vi "Modbus_spy.vi"() -> ()   [LabVIEW 2012]
uses:
  Controls/MBA_data.ctl
  <vilib>/Instr/_visa.llb/VISA Configure Serial Port (Instr).vi
panel:
  in  "string":string
  out "MBA data":T1
  in  "Array":string[](array[string])
  in  "Стоп":bool
  out "substring":string
  out "error out":errorcluster
  in  "error in (no error)":errorcluster
  in  "flow control":u16(ring) items=["None"=0, "XON/XOFF"=1, "RTS/CTS"=2, "DTR/DSR"=4]
  in  "stop bits":u16(ring)=10 items=["1.0"=10, "1.5"=15, "2.0"=20]
  in  "parity":u16(ring)=1 items=["None", "Odd", "Even", "Mark", "Space"]
  in  "data bits":u16=8 min=5 max=8 step=1
  in  "VISA resource name":refnum<visa-resource-name>="COM1"
  in  "baud rate":u32=19200
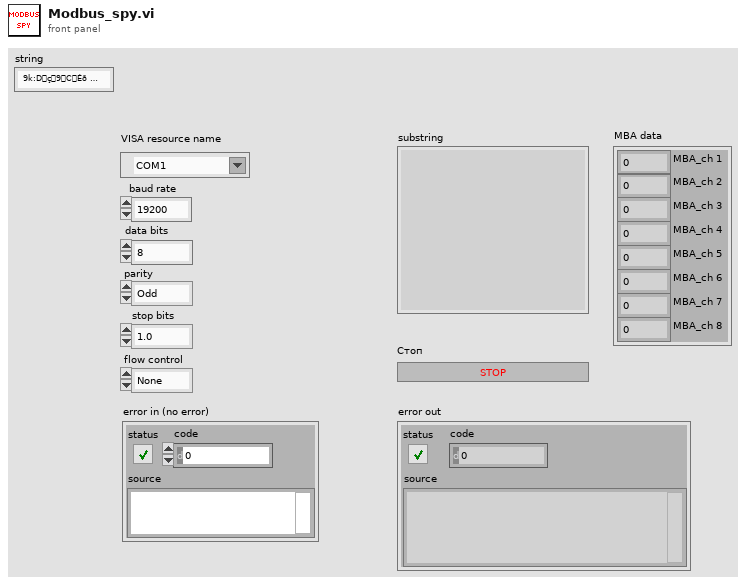
[diagram p1: front panel]
types:
  T1 = typedef "MBA_data.ctl" = cluster{"MBA_ch 1":dbl, "MBA_ch 2":dbl, "MBA_ch 3":dbl, "MBA_ch 4":dbl, "MBA_ch 5":dbl, "MBA_ch 6":dbl, "MBA_ch 7":dbl, "MBA_ch 8":dbl}
  T2 = cluster{"MBA_ch 1":dbl, "MBA_ch 2":dbl, "MBA_ch 3":dbl, "MBA_ch 4":dbl, "MBA_ch 5":dbl, "MBA_ch 6":dbl, "MBA_ch 7":dbl, "MBA_ch 8":dbl}
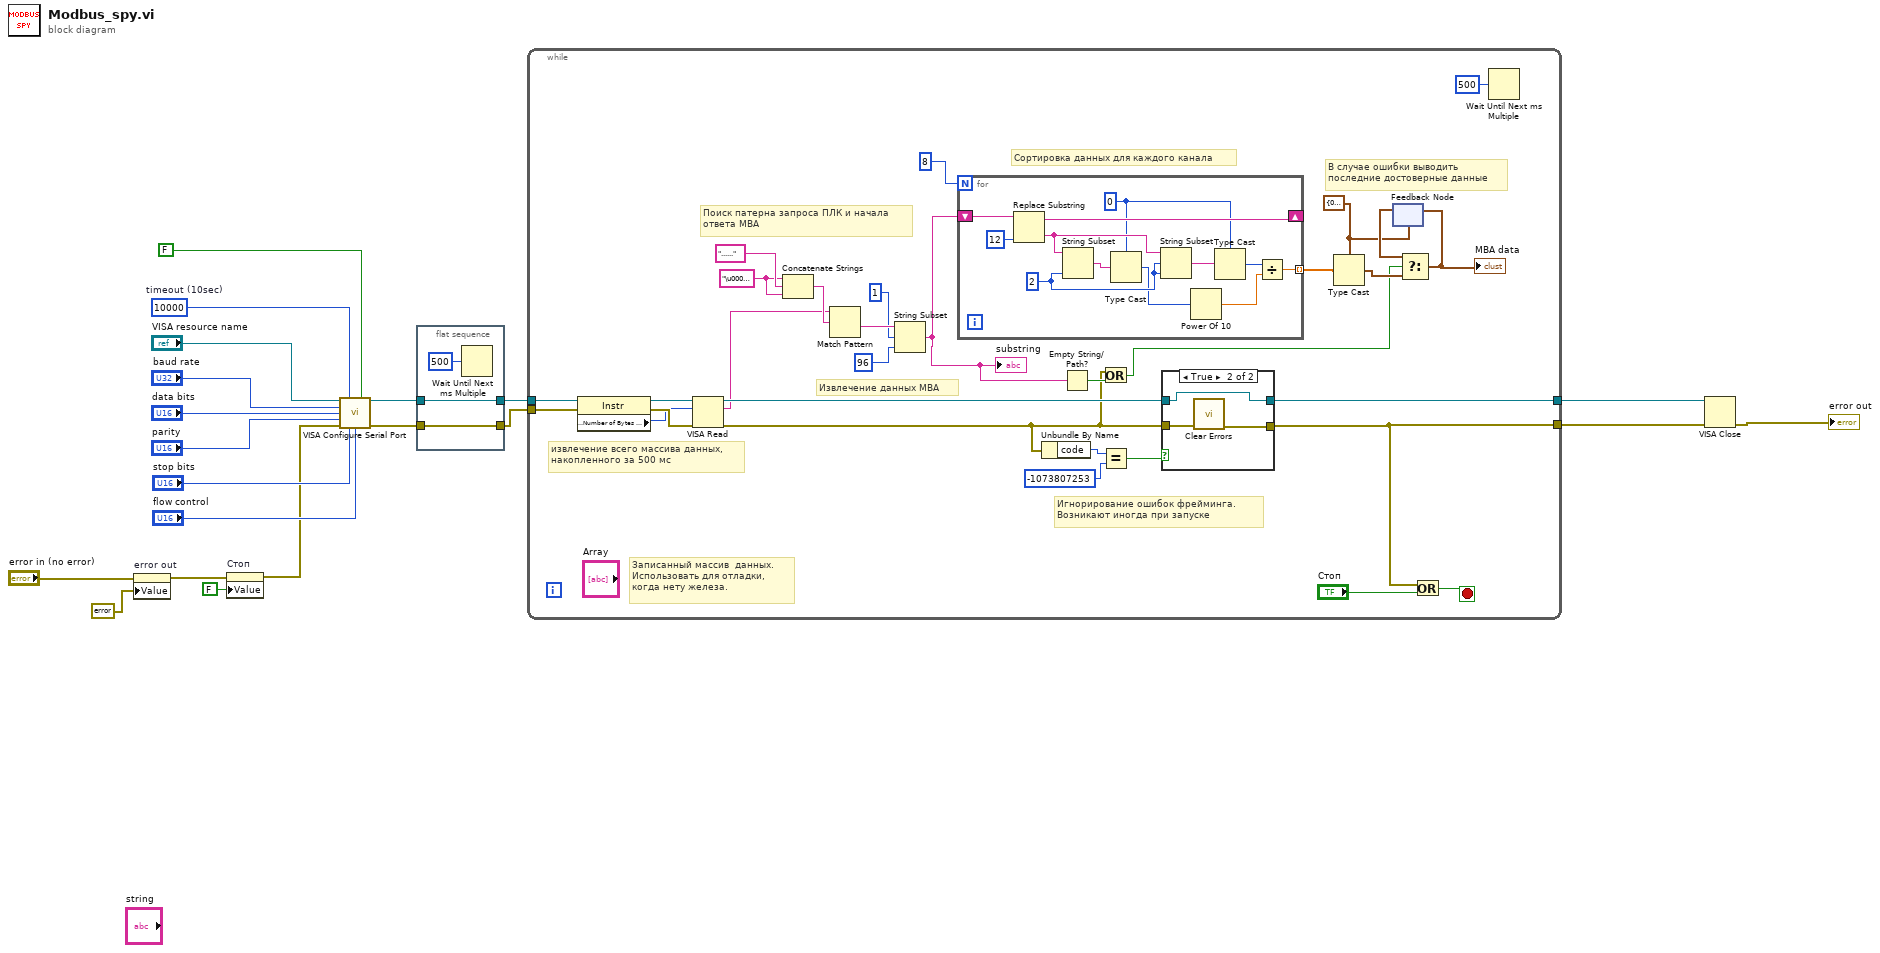
[diagram p0: block diagram]
diagram:
  w16 = u32 10000  # timeout (10sec)
  n1 = property on="error out" class="Clust (strict)"(error in="error in (no error)", "Value"=errorcluster {"status"=FALSE, "code"=0, "source"=""} ("error in (no error)")) -> (error out=w3:errorcluster)  [unwired: 1 in, 1 out]
  n2 = property on="Стоп" class="Bool (strict)"(error in=w3, "Value"=FALSE ("Стоп")) -> (error out=w6:errorcluster)  [unwired: 1 in, 1 out]
  n3 = call-poly "VISA Configure Serial Port"("VISA resource name"="VISA resource name", "timeout (10sec)"=w16, "Enable Termination\nChar (T)"=FALSE ("Enable Termination\nChar (T)"), "baud rate (9600)"="baud rate", "data bits (8)"="data bits", "parity (0:none)"="parity", "error in (no error)"=w6, "stop bits (10: 1 bit)"="stop bits", "flow control (0:none)"="flow control") -> ("VISA resource name out"=w10:refnum<visa-resource-name>, "error out"=w8:errorcluster)  [unwired: 5 out]
  n4 = flat-sequence {
    tunnel: w10 -> [w22]
    tunnel: [w22] -> w9
    tunnel: w8 -> [w21]
    tunnel: [w21] -> w7
    frame #0 {
      n5 = Wait Until Next ms Multiple(millisecond multiple=u32 500) -> ()  [unwired: 1 out]
    }
  }
  n6 = while {
    tunnel: [w32] -> w20
    tunnel: w9 -> [w51]
    tunnel: w7 -> [w50]
    tunnel: [w39] -> w4
    stop <- w45 stop-if-true
    w29 = T2 {"MBA_ch 1"=0.0, "MBA_ch 2"=0.0, "MBA_ch 3"=0.0, "MBA_ch 4"=0.0, "MBA_ch 5"=0.0, "MBA_ch 6"=0.0, "MBA_ch 7"=0.0, "MBA_ch 8"=0.0} ("MBA data")
    w48 = "\u0002\u0003" ("string")
    # "В случае ошибки выводить \nпоследние достоверные данные"
    # "Записанный массив  данных.\nИспользовать для отладки,\nкогда нету железа."
    # "Сортировка данных для каждого канала"
    # "Извлечение данных МВА"
    # "Игнорирование ошибок фрейминга.\nВозникают иногда при запуске"
    # "Поиск патерна запроса ПЛК и начала\nответа МВА"
    # "извлечение всего массива данных,\nнакопленного за 500 мс"
    n7 = property class="Instr"(reference=w51, error in=w50) -> (reference out=w54:refnum<visa-resource-name>, error out=w53:errorcluster, "Serial Settings:Number of Bytes at Serial Port"=w52:u32)
    n8 = VISA Read(VISA resource name=w54, byte count=w52, error in (no error)=w53) -> (VISA resource name out=w40:refnum<visa-resource-name>, read buffer=w33:string, error out=w25:errorcluster)  [unwired: 1 out]
    n9 = Concatenate Strings(w48, "......" ("regular expression"), w48) -> (w47:string)
    n10 = Match Pattern(string=w33, regular expression=w47) -> (after substring=w38:string)  [unwired: 1 in, 3 out]
    n11 = String Subset(string=w38, offset (0)=1, length (rest)=96 ("length (len. of substring)")) -> (substring=w27:string)
    "substring" <- w27
    n12 = for {
      N: 8 -> [_]
      shift-right: [w64] -> _
      shift-left: w27 -> [w66]
      tunnel: [w55] -> w34 mode=indexing
      w59 = i16 0
      w62 = 2 ("length (rest)")
      n13 = Replace Substring(2:12 ("length (len. of substring)"), 5:w66) -> (0:w61:string, 1:w64:string)  [unwired: 2 in]
      n14 = String Subset(string=w61, length (rest)=w62) -> (substring=w63:string)  [unwired: 1 in]
      n15 = Type Cast(type=w59, x=w63) -> (*(type *) &x=w57:i16)
      n16 = String Subset(string=w61, offset (0)=w62, length (rest)=w62) -> (substring=w60:string)
      n17 = Power Of 10(x=w57) -> (10^x=w56:dbl)
      n18 = Type Cast(type=w59, x=w60) -> (*(type *) &x=w58:i16)
      n19 = Divide(x=w58, y=w56) -> (x/y=w55:dbl)
    }
    n20 = Unbundle By Name(w25) -> ("code"=w43:i32)
    n21 = Empty String/Path?(string/path=w27) -> (empty?=w26:bool)
    n22 = Or(x=w25, y=w26) -> (x .or. y?=w24:bool)
    n23 = Equal?(x=w43, y=-1073807253) -> (x = y?=w41:bool)
    n24 = case shown="True" w41 {
      tunnel: w25 -> [w68 w71]
      tunnel: [w68 w70] -> w32
      tunnel: w40 -> [w67 w69]
      tunnel: [w67 w69] -> w39
      frame False {
      }
      frame True {
        n25 = call <vilib>:"Clear Errors.vi"("error in (no error)"=w71) -> ("error out"=w70:errorcluster)  [unwired: 6 in]
      }
    }
    n26 = Type Cast(type=w29, x=w34) -> (*(type *) &x=w31:T2)
    n27 = feedback #1(w29) -> (w30:T2)
    n28 = Select(t=w30, s=w24, f=w31) -> (s? t:f=w28:T2)
    "MBA data" <- w28
    n29 = feedback-in #1(w28) -> ()
    n30 = Or(x=w32, y="Стоп") -> (x .or. y?=w45:bool)
    n31 = Wait Until Next ms Multiple(millisecond multiple=u32 500) -> ()  [unwired: 1 out]
  }
  n32 = VISA Close(VISA resource name=w4, error in (no error)=w20) -> (error out=→"error out":errorcluster)
